vi "Get Hierarchical Names and Paths.vi"(7 "Parent Class":refnum<class>, 8 "error in (no error)":errorcluster, 10 "Class References":refnum<vi>[](array[refnum])) -> (0 "error out":errorcluster, 1 "Paths":path[](array[path]), 2 "Names":string[](array[string]))   [LabVIEW 2020, in "Process Generation.lvlib" / "New Class Dialog.lvclass"]
uses:
  New Class Dialog.lvclass
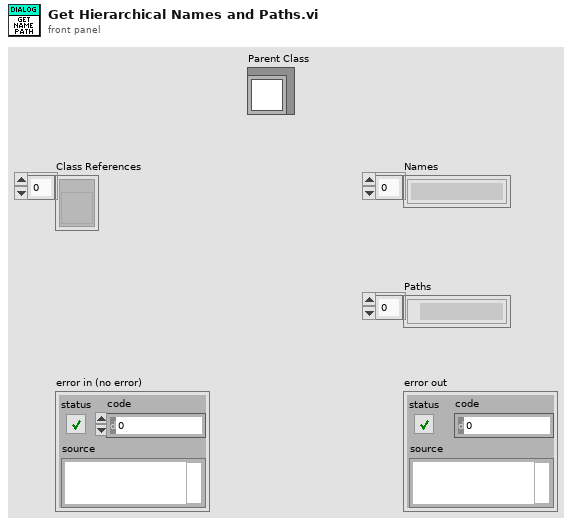
[diagram p1: front panel]
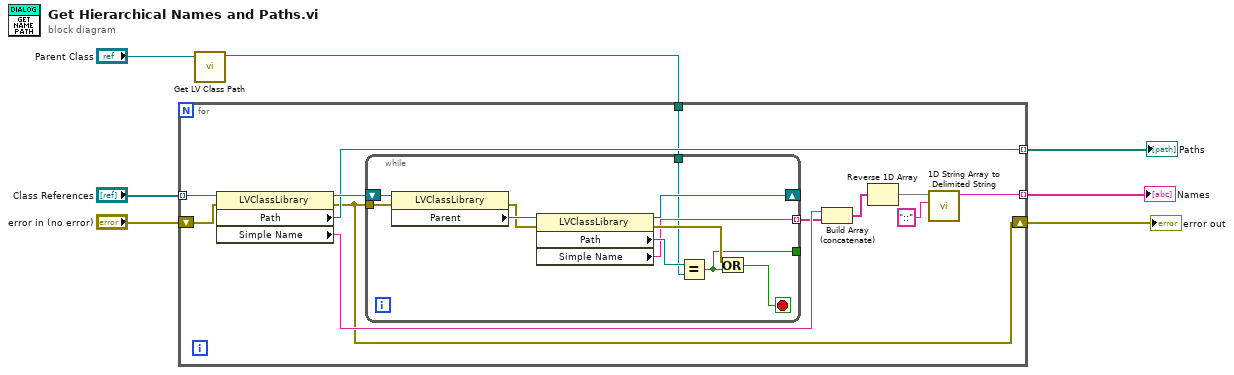
[diagram p0: block diagram]
diagram:
  n1 = call <vilib>:"Get LV Class Path.vi"("object"="Parent Class") -> ("class path"=w1:path)  [unwired: 9 in, 1 out]
  n2 = for {
    tunnel: "Class References" -> [w19] mode=indexing
    shift-right: [w9] -> w5
    shift-left: "error in (no error)" -> [w17]
    tunnel: [w11] -> w6 mode=indexing
    tunnel: [w10] -> w7 mode=indexing
    tunnel: w1 -> [w8]
    n3 = property class="LVClassLibrary"(reference=w19, error in=w17) -> (reference out=w18:refnum<vi>, error out=w9:errorcluster, "Path"=w10:path, "Simple Name"=w13:string)
    n4 = while {
      tunnel: w9 -> [w26]
      tunnel: [w23] -> w12 mode=indexing
      tunnel: [w22] -> _
      shift-right: [w21] -> _
      shift-left: w18 -> [w30]
      tunnel: w8 -> [w20]
      stop <- w24 stop-if-true
      n5 = property class="LVClassLibrary"(reference=w30, error in=w26) -> (error out=w27:errorcluster, "Parent"=w29:refnum<vi>)  [unwired: 1 out]
      n6 = property class="LVClassLibrary"(reference=w29, error in=w27) -> (reference out=w21:refnum<vi>, error out=w25:errorcluster, "Path"=w28:path, "Simple Name"=w23:string)
      n7 = Equal?(x=w28, y=w20) -> (x = y?=w22:bool)
      n8 = Or(x=w25, y=w22) -> (x .or. y?=w24:bool)
    }
    n9 = Build Array (concatenate)(w13, w12) -> (w16:string[])
    n10 = Reverse 1D Array(array=w16) -> (reversed array=w15:string[])
    n11 = call <vilib>:"1D String Array to Delimited String.vi"("delimiter"="::", "string array"=w15) -> ("delimited string"=w11:string)  [unwired: 9 in]
  }
  "error out" <- w5
  "Names" <- w6
  "Paths" <- w7
